vi "rcpacini_l_inline_subvi.vi"(6 "Variant in":variant, 7 "Shift Pressed?":bool, 8 "error in (no error)":errorcluster, 10 "QD Combo Box Ref":refnum<vi>, 11 "QD Launch VI Ref":refnum<vi>) -> (0 "error out":errorcluster, 4 "Variant out":variant)   [LabVIEW 2019]
doc: "Inline the selected SubVI into the current block diagram. Ctrl-Shift wraps the content in a sequence structure.\n\nCreated by: Ryan Pacini\n\nDefault Shortcut - [L]"
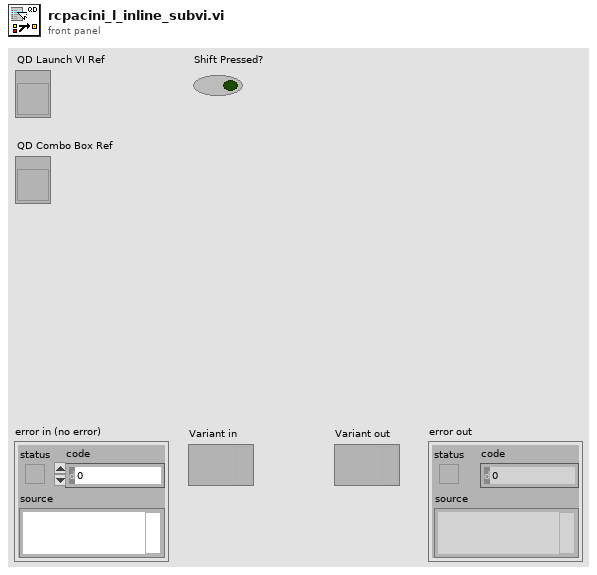
[diagram p1: front panel]
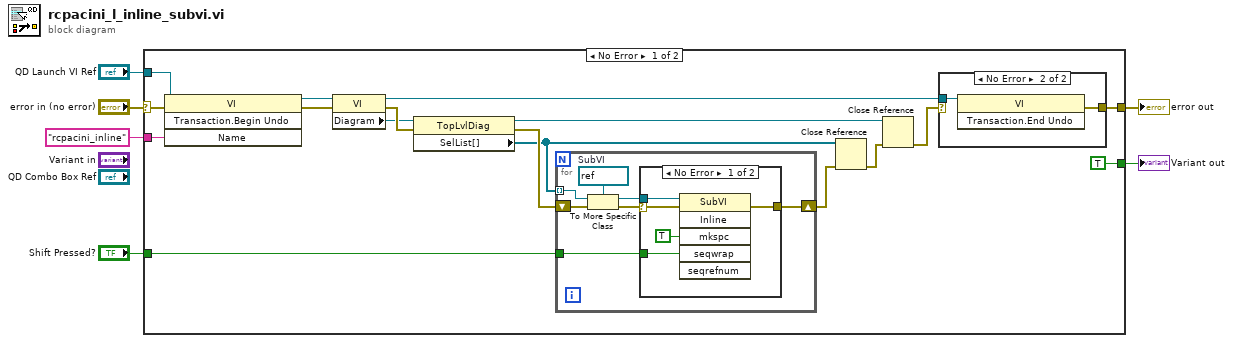
[diagram p0: block diagram]
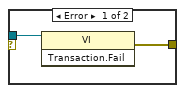
[diagram p3: hidden frame]
diagram:
  n1 = case shown="No Error" "error in (no error)" {
    selector: "error in (no error)" -> [w23 w40]
    tunnel: [w22 w40] -> w2
    tunnel: "QD Launch VI Ref" -> [w19 _]
    tunnel: "rcpacini_inline" ("Undo Name") -> [w21 _]
    tunnel: [TRUE _] -> w3
    tunnel: "Shift Pressed?" -> [w10 _]
    frame No Error {
      n2 = invoke class="VI" method="Transaction.Begin Undo"(reference=w19, error in=w23, "Name"=w21) -> (reference out=w17:refnum<vi>, error out=w18:errorcluster)  [unwired: 1 in, 2 out]
      n3 = property class="VI"(reference=w17, error in=w18) -> (reference out=w7:refnum<vi>, error out=w15:errorcluster, "Diagram"=w9:refnum<vi>)
      n4 = property class="TopLvlDiag"(reference=w9, error in=w15) -> (reference out=w8:refnum<vi>, error out=w14:errorcluster, "SelList[]"=w12:refnum<vi>[])
      n5 = for {
        shift-right: [w28] -> w13
        shift-left: w14 -> [w30]
        tunnel: w12 -> [w25] mode=indexing
        tunnel: w10 -> [w24]
        w29 = refnum<vi> refnum  # SubVI
        n6 = To More Specific Class(target class=w29, reference=w25, error in=w30) -> (specific class reference=w27:refnum<vi>, error out=w26:errorcluster)
        n7 = case shown="No Error" w26 {
          selector: w26 -> [w32 _]
          tunnel: [w35 _] -> w28
          tunnel: w27 -> [w33 _]
          tunnel: w24 -> [w31 _]
          frame No Error {
            n8 = invoke class="SubVI" method="Inline"(reference=w33, error in=w32, "mkspc"=TRUE ("Make Space in Block Diagram"), "seqwrap"=w31) -> (error out=w35:errorcluster)  [unwired: 2 in, 5 out]
          }
          frame Error {
          }
        }
      }
      n9 = Close Reference(reference=w12, error in (no error)=w13) -> (error out=w11:errorcluster)
      n10 = Close Reference(reference=w8, error in (no error)=w11) -> (error out=w16:errorcluster)
      n11 = case shown="No Error" w16 {
        tunnel: w7 -> [w36 w38]
        tunnel: [w37 w39] -> w22
        frame Error {
          n12 = invoke class="VI" method="Transaction.Fail"(reference=w36) -> (error out=w37:errorcluster)  [unwired: 2 in, 2 out]
        }
        frame No Error {
          n13 = invoke class="VI" method="Transaction.End Undo"(reference=w38) -> (error out=w39:errorcluster)  [unwired: 2 in, 2 out]
        }
      }
    }
    frame Error {
    }
  }
  "error out" <- w2
  "Variant out" <- w3
